vi "assignment - client.vi"() -> ()   [LabVIEW 2020]
panel:
  out "Login":bool=TRUE
  in  "Invalid":bool
  in  "stop":bool
  in  "Tab Control":T1(tab)
  in  "Enter":bool
  in  "0":bool
  in  "Reset":bool
  out "Instruction":string
  in  "9":bool
  in  "8":bool
  in  "7":bool
  in  "6":bool
  in  "5":bool
  in  "4":bool
  in  "3":bool
  in  "2":bool
  in  "1":bool
  out "PIN":string
  out "Verification":bool
  out "Time Stamp":timestamp format="%<%X\n%x>T"
  in  "Vacation mode":bool
  in  "Living Room":bool
  in  "Bedroom 1":bool
  in  "Bedroom 2":bool
  in  "Laundry 1":bool
  in  "Laundry 2":bool
  in  "Laundry 3":bool
  in  "Laundry 4":bool
  in  "Bathroom 1":bool
  in  "Bathroom 2":bool
  in  "Kitchen":bool
  in  "Dining":bool
  in  "Master":bool
  in  "Dining":dbl(knob) scale=0.0..255.0
  in  "Kitchen":dbl(knob) scale=0.0..255.0
  in  "Bathroom 2":dbl(knob) scale=0.0..255.0
  in  "Laundry 3":dbl(knob) scale=0.0..255.0
  in  "Bedroom 2":dbl(knob) scale=0.0..255.0
  in  "Bathroom 1":dbl(knob) scale=0.0..255.0
  in  "Laundry 2":dbl(knob) scale=0.0..255.0
  in  "Bedroom 1":dbl(knob) scale=0.0..255.0
  in  "Laundry 4":dbl(knob) scale=0.0..255.0
  in  "Laundry 1":dbl(knob) scale=0.0..255.0
  in  "Living Room":dbl(knob) scale=0.0..255.0
  in  "Bedroom 2":bool
  in  "Bedroom 1":bool
  in  "Master 2":bool
  in  "Automation":bool
  in  "Back":bool
  in  "Bathroom 2":bool
  in  "Laundry 4":bool
  in  "Laundry 2":bool
  in  "Laundry 1":bool
  in  "Bedroom 2":bool
  in  "Bedroom 1":bool
  in  "Front":bool
  in  "Master 3":bool
  in  "VolUp":bool
  in  "Stop":bool
  in  "Channel 2":bool
  in  "Channel 1":bool
  in  "VolDown":bool
  in  "FRwd":bool
  in  "Ffwd":bool
  in  "Pause":bool
  in  "Play":bool
  in  "Power":bool
  in  "Mute":bool
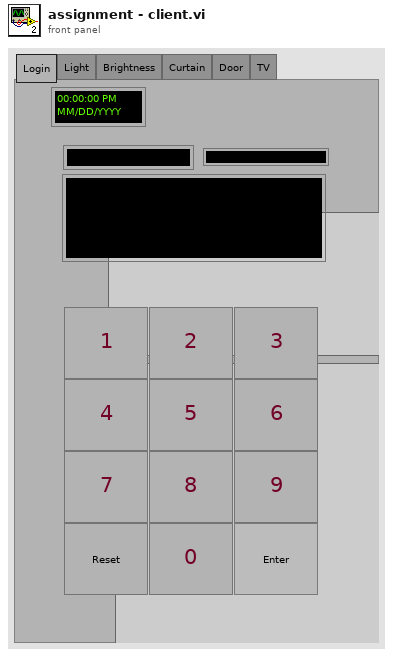
[diagram p1: front panel]
types:
  T1 = enum32{"Login", "Light", "Brightness", "Curtain", "Door", "TV"}
  T2 = enum32{"Page Enabled", "Page Disabled", "Page Disabled & Grayed"}
  T3 = enum8{"Enabled", "Disabled", "Disabled and Grayed Out"}
  T4 = enum32{"Invalid", "Standard", "Closed", "Hidden", "Minimized", "Maximized"}
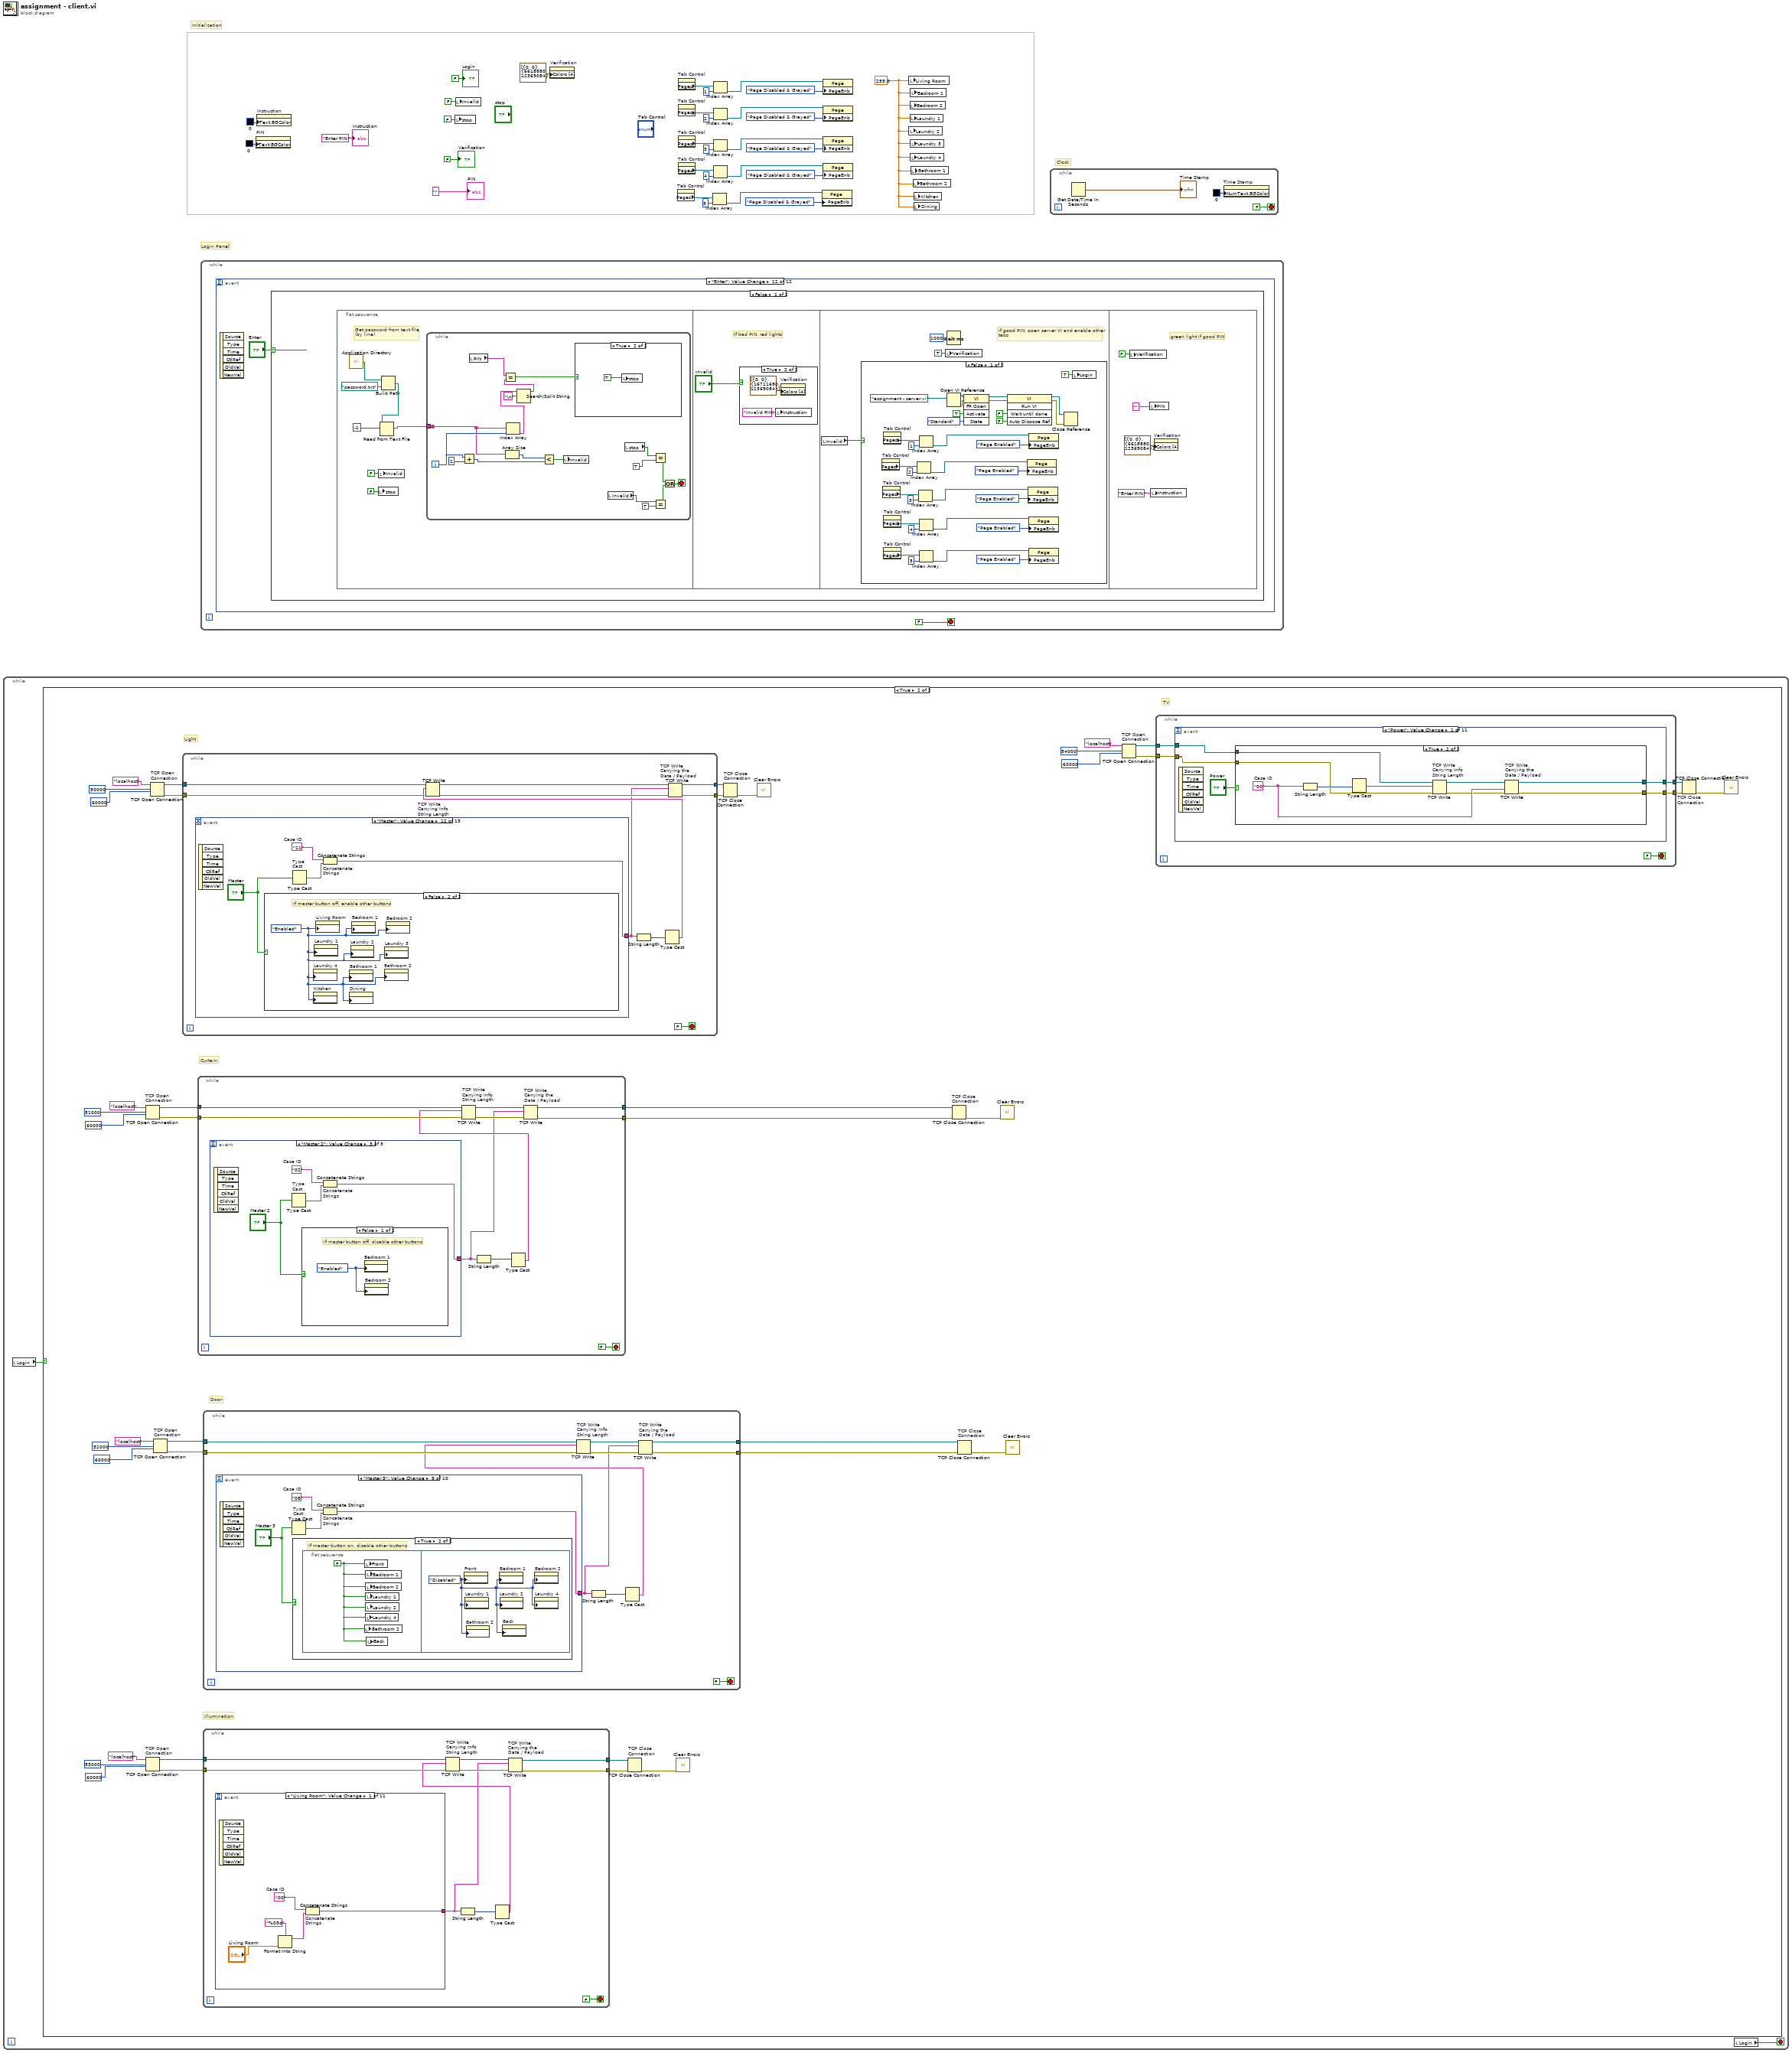
[diagram p0: block diagram]
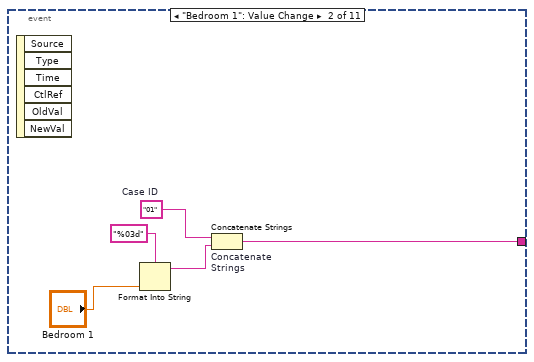
[diagram p3: hidden frame]
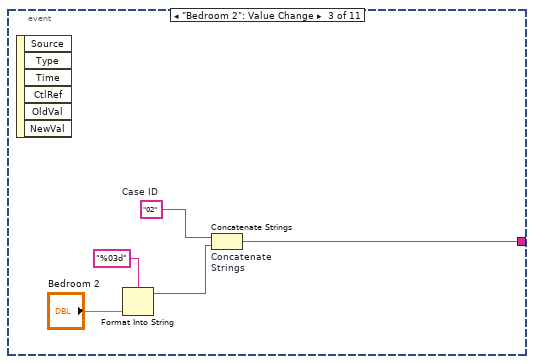
[diagram p4: hidden frame]
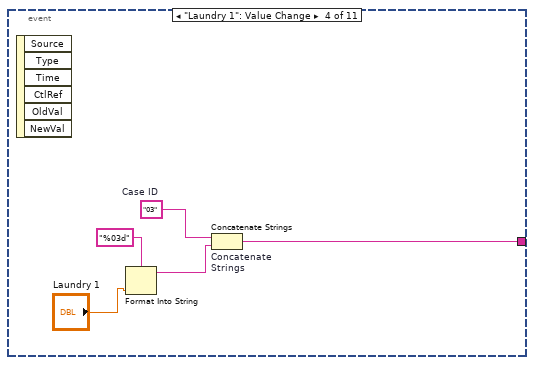
[diagram p5: hidden frame]
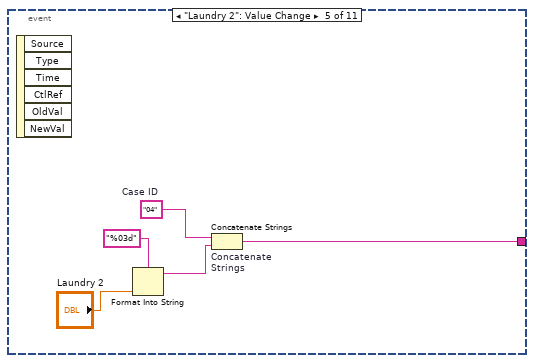
[diagram p6: hidden frame]
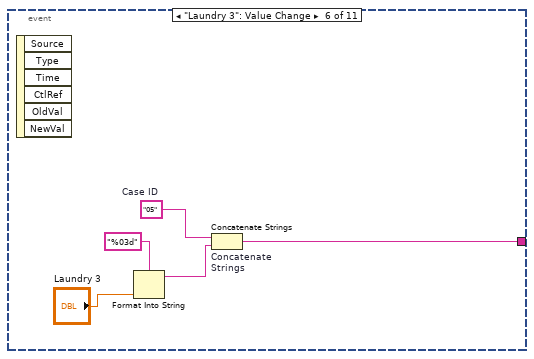
[diagram p7: hidden frame]
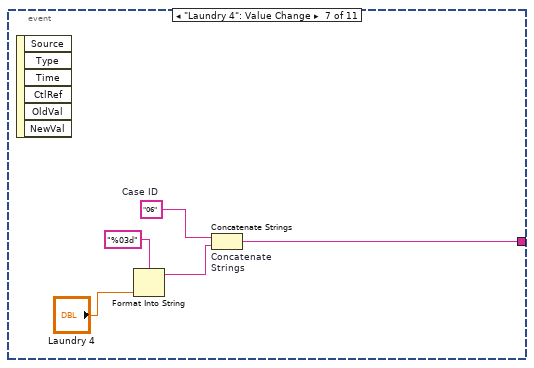
[diagram p8: hidden frame]
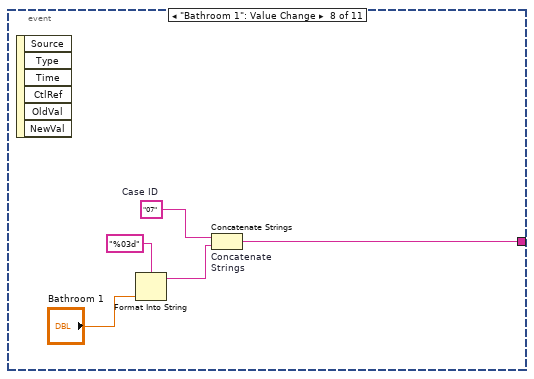
[diagram p9: hidden frame]
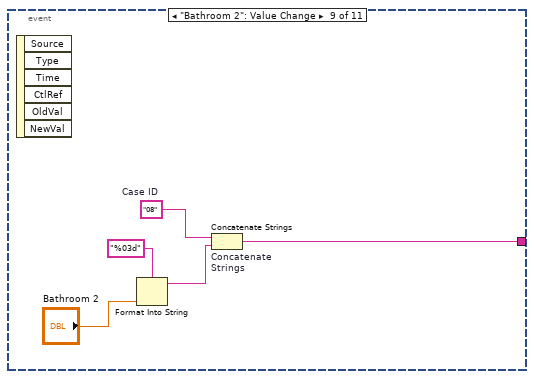
[diagram p10: hidden frame]
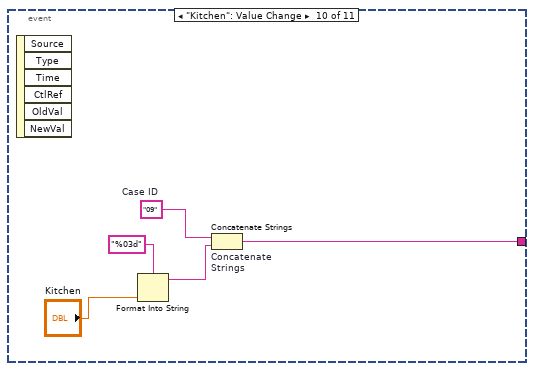
[diagram p11: hidden frame]
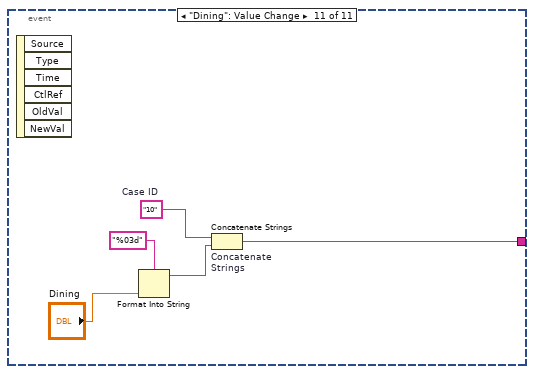
[diagram p12: hidden frame]
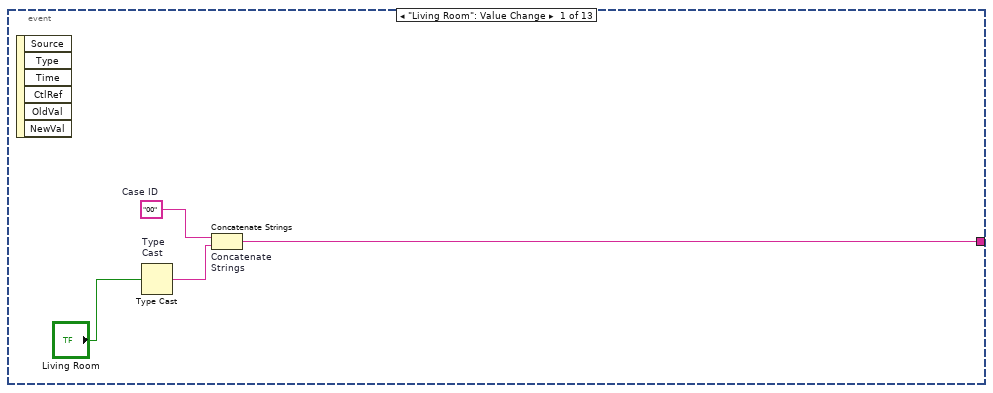
[diagram p13: hidden frame]
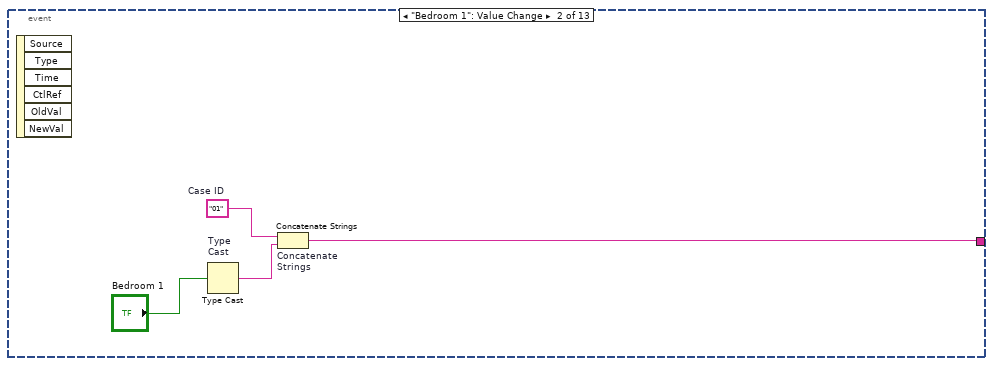
[diagram p14: hidden frame]
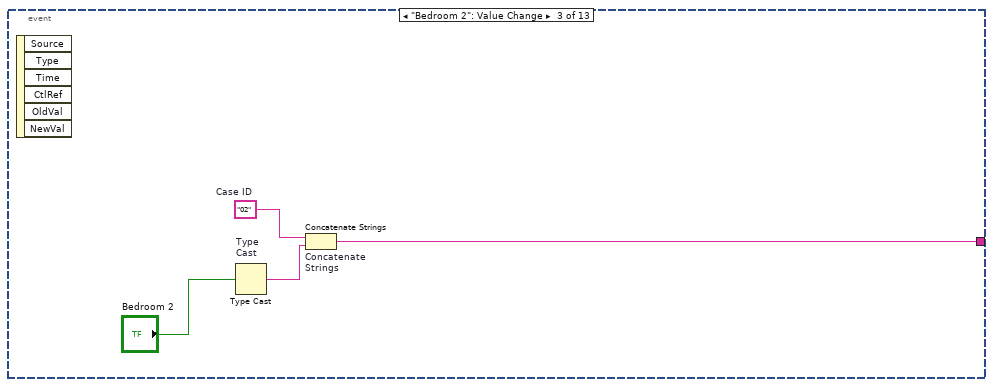
[diagram p15: hidden frame]
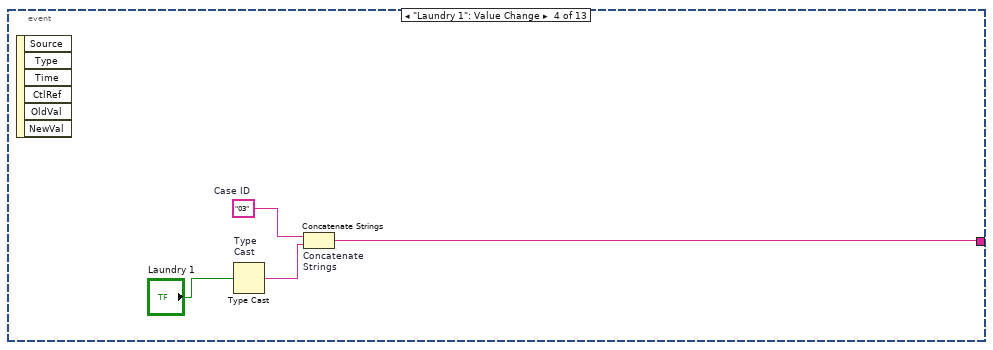
[diagram p16: hidden frame]
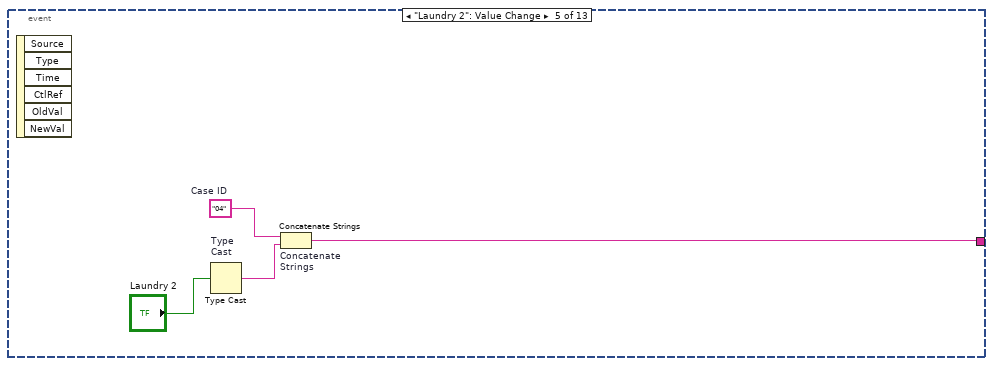
[diagram p17: hidden frame]
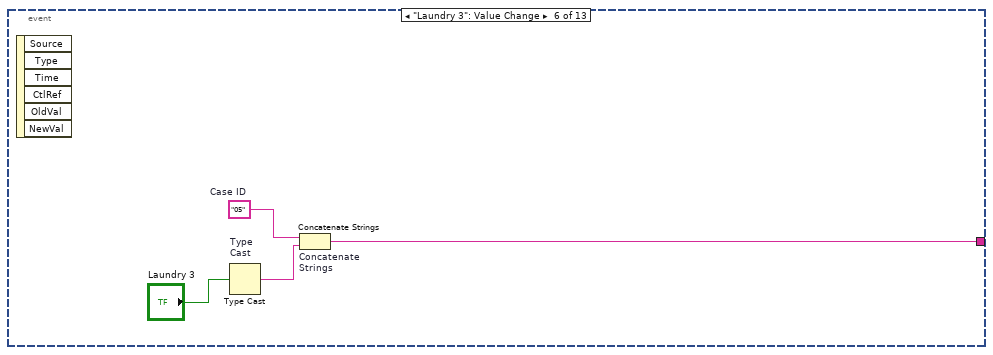
[diagram p18: hidden frame]
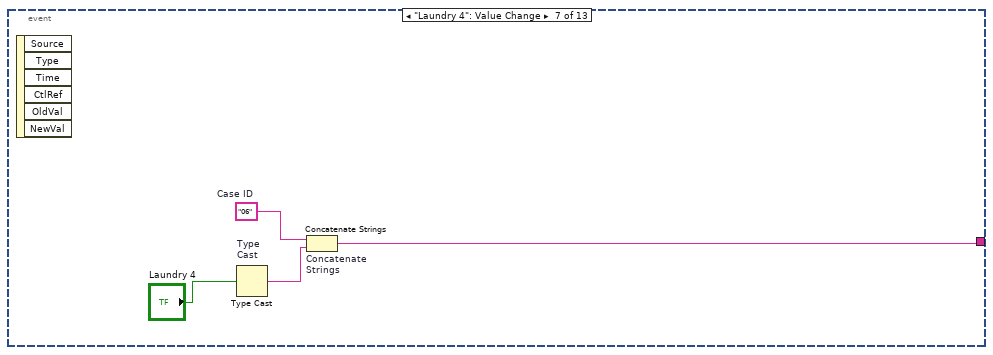
[diagram p19: hidden frame]
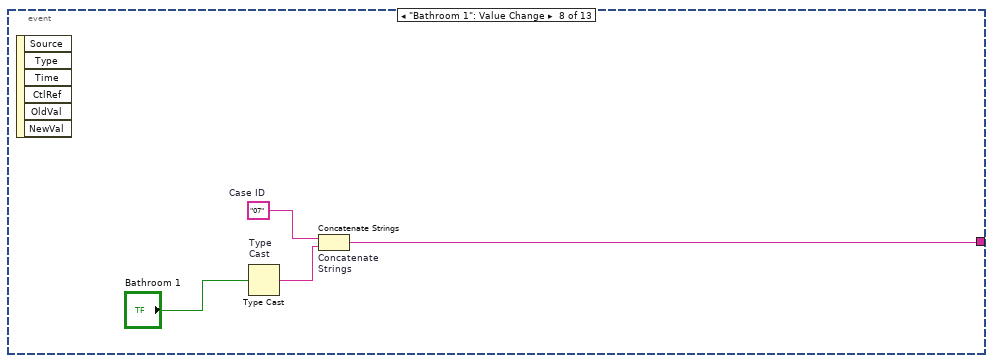
[diagram p20: hidden frame]
diagram:
  w21 = 255.0 ("Living Room")
  # "Clock"
  # "Initialization"
  # "Login Panel"
  n1 = while {
    stop <- w31 stop-if-true
    n2 = local read "Login"() -> (w32:bool)
    n3 = case shown="True" w32 {
      frame False {
      }
      frame True {
        # "TV"
        # "Illumination"
        # "Door"
        # "Curtain"
        # "Light"
        n4 = TCP Open Connection "TCP Open\nConnection"(address="localhost", remote port or service name=u16 51000, timeout ms (60000)=60000) -> (connection ID=w61:refnum<k5>, error out=w60:errorcluster)  [unwired: 2 in]
        n5 = TCP Open Connection "TCP Open\nConnection"(address="localhost", remote port or service name=u16 53000, timeout ms (60000)=60000) -> (connection ID=w33:refnum<k5>, error out=w34:errorcluster)  [unwired: 2 in]
        n6 = TCP Open Connection "TCP Open\nConnection"(address="localhost", remote port or service name=u16 50000, timeout ms (60000)=60000) -> (connection ID=w41:refnum<k5>, error out=w42:errorcluster)  [unwired: 2 in]
        n7 = TCP Open Connection "TCP Open\nConnection"(address="localhost", remote port or service name=u16 52000, timeout ms (60000)=60000) -> (connection ID=w53:refnum<k5>, error out=w52:errorcluster)  [unwired: 2 in]
        n8 = while {
          tunnel: [w141] -> w48
          tunnel: [w140] -> w47
          tunnel: w42 -> [w139]
          tunnel: w41 -> [w138]
          stop <- FALSE stop-if-true
          n9 = event shown="[11] \"Master\": Value Change" {
            selector: _ -> [_ _ _ _ _ _ _ _ _ _ _ _ _]
            dyn-events: _ -> [_ _ _ _ _ _ _ _ _ _ _ _ _]
            timeout: _ -> [_ _ _ _ _ _ _ _ _ _ _ _ _]
            tunnel: [w148 w152 w156 w161 w164 w168 w172 w176 w180 w184 w188 w193 w200] -> w142
            event "Living Room": Value Change {
              w149 = "00"  # Case ID
              n10 = event-data() -> ()  [unwired: 1 in, 6 out]
              n11 = Type Cast "Type \nCast"(x="Living Room") -> (*(type *) &x=w150:string)  [unwired: 1 in]
              n12 = Concatenate Strings "Concatenate \nStrings"(w149, w150) -> (w148:string)
            }
            event "Bedroom 1": Value Change {
              w154 = "01"  # Case ID
              n13 = event-data() -> ()  [unwired: 1 in, 6 out]
              n14 = Type Cast "Type \nCast"(x="Bedroom 1") -> (*(type *) &x=w155:string)  [unwired: 1 in]
              n15 = Concatenate Strings "Concatenate \nStrings"(w154, w155) -> (w152:string)
            }
            event "Bedroom 2": Value Change {
              w158 = "02"  # Case ID
              n16 = event-data() -> ()  [unwired: 1 in, 6 out]
              n17 = Type Cast "Type \nCast"(x="Bedroom 2") -> (*(type *) &x=w159:string)  [unwired: 1 in]
              n18 = Concatenate Strings "Concatenate \nStrings"(w158, w159) -> (w156:string)
            }
            event "Laundry 1": Value Change {
              w162 = "03"  # Case ID
              n19 = event-data() -> ()  [unwired: 1 in, 6 out]
              n20 = Type Cast "Type \nCast"(x="Laundry 1") -> (*(type *) &x=w163:string)  [unwired: 1 in]
              n21 = Concatenate Strings "Concatenate \nStrings"(w162, w163) -> (w161:string)
            }
            event "Laundry 2": Value Change {
              w166 = "04"  # Case ID
              n22 = event-data() -> ()  [unwired: 1 in, 6 out]
              n23 = Type Cast "Type \nCast"(x="Laundry 2") -> (*(type *) &x=w167:string)  [unwired: 1 in]
              n24 = Concatenate Strings "Concatenate \nStrings"(w166, w167) -> (w164:string)
            }
            event "Laundry 3": Value Change {
              w170 = "05"  # Case ID
              n25 = event-data() -> ()  [unwired: 1 in, 6 out]
              n26 = Type Cast "Type \nCast"(x="Laundry 3") -> (*(type *) &x=w171:string)  [unwired: 1 in]
              n27 = Concatenate Strings "Concatenate \nStrings"(w170, w171) -> (w168:string)
            }
            event "Laundry 4": Value Change {
              w174 = "06"  # Case ID
              n28 = event-data() -> ()  [unwired: 1 in, 6 out]
              n29 = Type Cast "Type \nCast"(x="Laundry 4") -> (*(type *) &x=w175:string)  [unwired: 1 in]
              n30 = Concatenate Strings "Concatenate \nStrings"(w174, w175) -> (w172:string)
            }
            event "Bathroom 1": Value Change {
              w178 = "07"  # Case ID
              n31 = event-data() -> ()  [unwired: 1 in, 6 out]
              n32 = Type Cast "Type \nCast"(x="Bathroom 1") -> (*(type *) &x=w179:string)  [unwired: 1 in]
              n33 = Concatenate Strings "Concatenate \nStrings"(w178, w179) -> (w176:string)
            }
            event "Bathroom 2": Value Change {
              w182 = "08"  # Case ID
              n34 = event-data() -> ()  [unwired: 1 in, 6 out]
              n35 = Type Cast "Type \nCast"(x="Bathroom 2") -> (*(type *) &x=w183:string)  [unwired: 1 in]
              n36 = Concatenate Strings "Concatenate \nStrings"(w182, w183) -> (w180:string)
            }
            event "Kitchen": Value Change {
              w186 = "09"  # Case ID
              n37 = event-data() -> ()  [unwired: 1 in, 6 out]
              n38 = Type Cast "Type \nCast"(x="Kitchen") -> (*(type *) &x=w187:string)  [unwired: 1 in]
              n39 = Concatenate Strings "Concatenate \nStrings"(w186, w187) -> (w184:string)
            }
            event "Dining": Value Change {
              w190 = "10"  # Case ID
              n40 = event-data() -> ()  [unwired: 1 in, 6 out]
              n41 = Type Cast "Type \nCast"(x="Dining") -> (*(type *) &x=w191:string)  [unwired: 1 in]
              n42 = Concatenate Strings "Concatenate \nStrings"(w190, w191) -> (w188:string)
            }
            event "Master": Value Change {
              w194 = "11"  # Case ID
              n43 = event-data() -> ()  [unwired: 1 in, 6 out]
              n44 = case shown="False" "Master" {
                frame True {
                  # "If master button ON, disable other buttons"
                  n45 = flat-sequence {
                    frame #0 {
                      w196 = FALSE ("Living Room")
                      n46 = local write "Living Room"(w196) -> ()
                      n47 = local write "Laundry 1"(w196) -> ()
                      n48 = local write "Laundry 4"(w196) -> ()
                      n49 = local write "Kitchen"(w196) -> ()
                      n50 = local write "Bedroom 1"(w196) -> ()
                      n51 = local write "Bathroom 1"(w196) -> ()
                      n52 = local write "Laundry 2"(w196) -> ()
                      n53 = local write "Dining"(w196) -> ()
                      n54 = local write "Bedroom 2"(w196) -> ()
                      n55 = local write "Laundry 3"(w196) -> ()
                      n56 = local write "Bathroom 2"(w196) -> ()
                    }
                    frame #1 {
                      w197 = T3."Disabled" ("Disabled")
                      n57 = property on="Laundry 4" class="Bool (strict)"("DisabledEnum"=w197) -> ()  [unwired: 2 in, 2 out]
                      n58 = property on="Kitchen" class="Bool (strict)"("DisabledEnum"=w197) -> ()  [unwired: 2 in, 2 out]
                      n59 = property on="Laundry 1" class="Bool (strict)"("DisabledEnum"=w197) -> ()  [unwired: 2 in, 2 out]
                      n60 = property on="Living Room" class="Bool (strict)"("DisabledEnum"=w197) -> ()  [unwired: 2 in, 2 out]
                      n61 = property on="Bathroom 1" class="Bool (strict)"("DisabledEnum"=w197) -> ()  [unwired: 2 in, 2 out]
                      n62 = property on="Dining" class="Bool (strict)"("DisabledEnum"=w197) -> ()  [unwired: 2 in, 2 out]
                      n63 = property on="Laundry 2" class="Bool (strict)"("DisabledEnum"=w197) -> ()  [unwired: 2 in, 2 out]
                      n64 = property on="Bedroom 1" class="Bool (strict)"("DisabledEnum"=w197) -> ()  [unwired: 2 in, 2 out]
                      n65 = property on="Bathroom 2" class="Bool (strict)"("DisabledEnum"=w197) -> ()  [unwired: 2 in, 2 out]
                      n66 = property on="Laundry 3" class="Bool (strict)"("DisabledEnum"=w197) -> ()  [unwired: 2 in, 2 out]
                      n67 = property on="Bedroom 2" class="Bool (strict)"("DisabledEnum"=w197) -> ()  [unwired: 2 in, 2 out]
                    }
                  }
                }
                frame False {
                  w198 = T3."Enabled" ("Disabled")
                  # "If master button off, enable other buttons"
                  n68 = property on="Laundry 4" class="Bool (strict)"("DisabledEnum"=w198) -> ()  [unwired: 2 in, 2 out]
                  n69 = property on="Kitchen" class="Bool (strict)"("DisabledEnum"=w198) -> ()  [unwired: 2 in, 2 out]
                  n70 = property on="Laundry 1" class="Bool (strict)"("DisabledEnum"=w198) -> ()  [unwired: 2 in, 2 out]
                  n71 = property on="Living Room" class="Bool (strict)"("DisabledEnum"=w198) -> ()  [unwired: 2 in, 2 out]
                  n72 = property on="Bathroom 1" class="Bool (strict)"("DisabledEnum"=w198) -> ()  [unwired: 2 in, 2 out]
                  n73 = property on="Dining" class="Bool (strict)"("DisabledEnum"=w198) -> ()  [unwired: 2 in, 2 out]
                  n74 = property on="Laundry 2" class="Bool (strict)"("DisabledEnum"=w198) -> ()  [unwired: 2 in, 2 out]
                  n75 = property on="Bedroom 1" class="Bool (strict)"("DisabledEnum"=w198) -> ()  [unwired: 2 in, 2 out]
                  n76 = property on="Bathroom 2" class="Bool (strict)"("DisabledEnum"=w198) -> ()  [unwired: 2 in, 2 out]
                  n77 = property on="Laundry 3" class="Bool (strict)"("DisabledEnum"=w198) -> ()  [unwired: 2 in, 2 out]
                  n78 = property on="Bedroom 2" class="Bool (strict)"("DisabledEnum"=w198) -> ()  [unwired: 2 in, 2 out]
                }
              }
              n79 = Type Cast "Type \nCast"(x="Master") -> (*(type *) &x=w195:string)  [unwired: 1 in]
              n80 = Concatenate Strings "Concatenate \nStrings"(w194, w195) -> (w193:string)
            }
            event "Vacation mode": Value Change {
              w201 = "12"  # Case ID
              n81 = event-data() -> ()  [unwired: 1 in, 6 out]
              n82 = Type Cast "Type \nCast"(x="Vacation mode") -> (*(type *) &x=w202:string)  [unwired: 1 in]
              n83 = Concatenate Strings "Concatenate \nStrings"(w201, w202) -> (w200:string)
            }
          }
          n84 = String Length(string=w142) -> (length=w146:i32)
          n85 = Type Cast(x=w146) -> (*(type *) &x=w145:string)  [unwired: 1 in]
          n86 = TCP Write "TCP Write\nCarrying Info\nString Length"(connection ID=w138, data in=w145, error in (no error)=w139) -> (connection ID out=w144:refnum<k5>, error out=w143:errorcluster)  [unwired: 1 in, 1 out]
          n87 = TCP Write "TCP Write\nCarrying the\nData / Payload"(connection ID=w144, data in=w142, error in (no error)=w143) -> (connection ID out=w141:refnum<k5>, error out=w140:errorcluster)  [unwired: 1 in, 1 out]
        }
        n88 = while {
          tunnel: w61 -> [w263]
          tunnel: w60 -> [w262]
          tunnel: [w257] -> w59
          tunnel: [w256] -> w58
          stop <- FALSE stop-if-true
          n89 = event shown="[2] \"Master 2\": Value Change" {
            selector: _ -> [_ _ _]
            dyn-events: _ -> [_ _ _]
            timeout: _ -> [_ _ _]
            tunnel: [w267 w271 w275] -> w258
            event "Bedroom 1": Value Change {
              w268 = "00"  # Case ID
              n90 = event-data() -> ()  [unwired: 1 in, 6 out]
              n91 = Type Cast "Type \nCast"(x="Bedroom 1") -> (*(type *) &x=w269:string)  [unwired: 1 in]
              n92 = Concatenate Strings "Concatenate \nStrings"(w268, w269) -> (w267:string)
            }
            event "Bedroom 2": Value Change {
              w272 = "01"  # Case ID
              n93 = event-data() -> ()  [unwired: 1 in, 6 out]
              n94 = Type Cast "Type \nCast"(x="Bedroom 2") -> (*(type *) &x=w273:string)  [unwired: 1 in]
              n95 = Concatenate Strings "Concatenate \nStrings"(w272, w273) -> (w271:string)
            }
            event "Master 2": Value Change {
              w276 = "02"  # Case ID
              n96 = event-data() -> ()  [unwired: 1 in, 6 out]
              n97 = Type Cast "Type \nCast"(x="Master 2") -> (*(type *) &x=w277:string)  [unwired: 1 in]
              n98 = case shown="False" "Master 2" {
                frame False {
                  w278 = T3."Enabled" ("Disabled")
                  # "If master button off, disable other buttons"
                  n99 = property on="Bedroom 1" class="Bool (strict)"("DisabledEnum"=w278) -> ()  [unwired: 2 in, 2 out]
                  n100 = property on="Bedroom 2" class="Bool (strict)"("DisabledEnum"=w278) -> ()  [unwired: 2 in, 2 out]
                }
                frame True {
                  # "If master button on, disable other buttons"
                  n101 = flat-sequence {
                    frame #0 {
                      w279 = FALSE ("Bedroom 1")
                      n102 = local write "Bedroom 1"(w279) -> ()
                      n103 = local write "Bedroom 2"(w279) -> ()
                    }
                    frame #1 {
                      w280 = T3."Disabled" ("Disabled")
                      n104 = property on="Bedroom 1" class="Bool (strict)"("DisabledEnum"=w280) -> ()  [unwired: 2 in, 2 out]
                      n105 = property on="Bedroom 2" class="Bool (strict)"("DisabledEnum"=w280) -> ()  [unwired: 2 in, 2 out]
                    }
                  }
                }
              }
              n106 = Concatenate Strings "Concatenate \nStrings"(w276, w277) -> (w275:string)
            }
          }
          n107 = String Length(string=w258) -> (length=w264:i32)
          n108 = Type Cast(x=w264) -> (*(type *) &x=w261:string)  [unwired: 1 in]
          n109 = TCP Write "TCP Write\nCarrying Info\nString Length"(connection ID=w263, data in=w261, error in (no error)=w262) -> (connection ID out=w260:refnum<k5>, error out=w259:errorcluster)  [unwired: 1 in, 1 out]
          n110 = TCP Write "TCP Write\nCarrying the\nData / Payload"(connection ID=w260, data in=w258, error in (no error)=w259) -> (connection ID out=w257:refnum<k5>, error out=w256:errorcluster)  [unwired: 1 in, 1 out]
        }
        n111 = while {
          tunnel: [w76] -> w40
          tunnel: [w75] -> w39
          tunnel: w34 -> [w74]
          tunnel: w33 -> [w73]
          stop <- FALSE stop-if-true
          n112 = event shown="[0] \"Living Room\": Value Change" {
            selector: _ -> [_ _ _ _ _ _ _ _ _ _ _]
            dyn-events: _ -> [_ _ _ _ _ _ _ _ _ _ _]
            timeout: _ -> [_ _ _ _ _ _ _ _ _ _ _]
            tunnel: [w86 w91 w96 w101 w106 w111 w116 w121 w126 w131 w136] -> w77
            event "Living Room": Value Change {
              w87 = "00"  # Case ID
              n113 = event-data() -> ()  [unwired: 1 in, 6 out]
              n114 = Format Into String "Format Into String"(format string="%03d", "Living Room") -> (resulting string=w83:string)  [unwired: 2 in, 1 out]
              n115 = Concatenate Strings "Concatenate \nStrings"(w87, w83) -> (w86:string)
            }
            event "Bedroom 1": Value Change {
              w92 = "01"  # Case ID
              n116 = event-data() -> ()  [unwired: 1 in, 6 out]
              n117 = Format Into String "Format Into String"(format string="%03d", "Bedroom 1") -> (resulting string=w88:string)  [unwired: 2 in, 1 out]
              n118 = Concatenate Strings "Concatenate \nStrings"(w92, w88) -> (w91:string)
            }
            event "Bedroom 2": Value Change {
              w97 = "02"  # Case ID
              n119 = event-data() -> ()  [unwired: 1 in, 6 out]
              n120 = Format Into String "Format Into String"(format string="%03d", "Bedroom 2") -> (resulting string=w93:string)  [unwired: 2 in, 1 out]
              n121 = Concatenate Strings "Concatenate \nStrings"(w97, w93) -> (w96:string)
            }
            event "Laundry 1": Value Change {
              w102 = "03"  # Case ID
              n122 = event-data() -> ()  [unwired: 1 in, 6 out]
              n123 = Format Into String "Format Into String"(format string="%03d", "Laundry 1") -> (resulting string=w98:string)  [unwired: 2 in, 1 out]
              n124 = Concatenate Strings "Concatenate \nStrings"(w102, w98) -> (w101:string)
            }
            event "Laundry 2": Value Change {
              w107 = "04"  # Case ID
              n125 = event-data() -> ()  [unwired: 1 in, 6 out]
              n126 = Format Into String "Format Into String"(format string="%03d", "Laundry 2") -> (resulting string=w103:string)  [unwired: 2 in, 1 out]
              n127 = Concatenate Strings "Concatenate \nStrings"(w107, w103) -> (w106:string)
            }
            event "Laundry 3": Value Change {
              w112 = "05"  # Case ID
              n128 = event-data() -> ()  [unwired: 1 in, 6 out]
              n129 = Format Into String "Format Into String"(format string="%03d", "Laundry 3") -> (resulting string=w108:string)  [unwired: 2 in, 1 out]
              n130 = Concatenate Strings "Concatenate \nStrings"(w112, w108) -> (w111:string)
            }
            event "Laundry 4": Value Change {
              w117 = "06"  # Case ID
              n131 = event-data() -> ()  [unwired: 1 in, 6 out]
              n132 = Format Into String "Format Into String"(format string="%03d", "Laundry 4") -> (resulting string=w113:string)  [unwired: 2 in, 1 out]
              n133 = Concatenate Strings "Concatenate \nStrings"(w117, w113) -> (w116:string)
            }
            event "Bathroom 1": Value Change {
              w122 = "07"  # Case ID
              n134 = event-data() -> ()  [unwired: 1 in, 6 out]
              n135 = Format Into String "Format Into String"(format string="%03d", "Bathroom 1") -> (resulting string=w118:string)  [unwired: 2 in, 1 out]
              n136 = Concatenate Strings "Concatenate \nStrings"(w122, w118) -> (w121:string)
            }
            event "Bathroom 2": Value Change {
              w127 = "08"  # Case ID
              n137 = event-data() -> ()  [unwired: 1 in, 6 out]
              n138 = Format Into String "Format Into String"(format string="%03d", "Bathroom 2") -> (resulting string=w123:string)  [unwired: 2 in, 1 out]
              n139 = Concatenate Strings "Concatenate \nStrings"(w127, w123) -> (w126:string)
            }
            event "Kitchen": Value Change {
              w132 = "09"  # Case ID
              n140 = event-data() -> ()  [unwired: 1 in, 6 out]
              n141 = Format Into String "Format Into String"(format string="%03d", "Kitchen") -> (resulting string=w128:string)  [unwired: 2 in, 1 out]
              n142 = Concatenate Strings "Concatenate \nStrings"(w132, w128) -> (w131:string)
            }
            event "Dining": Value Change {
              w137 = "10"  # Case ID
              n143 = event-data() -> ()  [unwired: 1 in, 6 out]
              n144 = Format Into String "Format Into String"(format string="%03d", "Dining") -> (resulting string=w133:string)  [unwired: 2 in, 1 out]
              n145 = Concatenate Strings "Concatenate \nStrings"(w137, w133) -> (w136:string)
            }
          }
          n146 = String Length(string=w77) -> (length=w81:i32)
          n147 = Type Cast(x=w81) -> (*(type *) &x=w80:string)  [unwired: 1 in]
          n148 = TCP Write "TCP Write\nCarrying Info\nString Length"(connection ID=w73, data in=w80, error in (no error)=w74) -> (connection ID out=w79:refnum<k5>, error out=w78:errorcluster)  [unwired: 1 in, 1 out]
          n149 = TCP Write "TCP Write\nCarrying the\nData / Payload"(connection ID=w79, data in=w77, error in (no error)=w78) -> (connection ID out=w76:refnum<k5>, error out=w75:errorcluster)  [unwired: 1 in, 1 out]
        }
        n150 = while {
          tunnel: w53 -> [w210]
          tunnel: w52 -> [w209]
          tunnel: [w204] -> w51
          tunnel: [w203] -> w50
          stop <- FALSE stop-if-true
          n151 = event shown="[8] \"Master 3\": Value Change" {
            selector: _ -> [_ _ _ _ _ _ _ _ _ _]
            dyn-events: _ -> [_ _ _ _ _ _ _ _ _ _]
            timeout: _ -> [_ _ _ _ _ _ _ _ _ _]
            tunnel: [w214 w218 w222 w226 w230 w234 w238 w242 w246 w253] -> w205
            event "Front": Value Change {
              w215 = "00"  # Case ID
              n152 = event-data() -> ()  [unwired: 1 in, 6 out]
              n153 = Type Cast "Type \nCast"(x="Front") -> (*(type *) &x=w216:string)  [unwired: 1 in]
              n154 = Concatenate Strings "Concatenate \nStrings"(w215, w216) -> (w214:string)
            }
            event "Bedroom 1": Value Change {
              w219 = "01"  # Case ID
              n155 = event-data() -> ()  [unwired: 1 in, 6 out]
              n156 = Type Cast "Type \nCast"(x="Bedroom 1") -> (*(type *) &x=w220:string)  [unwired: 1 in]
              n157 = Concatenate Strings "Concatenate \nStrings"(w219, w220) -> (w218:string)
            }
            event "Bedroom 2": Value Change {
              w223 = "02"  # Case ID
              n158 = event-data() -> ()  [unwired: 1 in, 6 out]
              n159 = Type Cast "Type \nCast"(x="Bedroom 2") -> (*(type *) &x=w224:string)  [unwired: 1 in]
              n160 = Concatenate Strings "Concatenate \nStrings"(w223, w224) -> (w222:string)
            }
            event "Laundry 1": Value Change {
              w227 = "03"  # Case ID
              n161 = event-data() -> ()  [unwired: 1 in, 6 out]
              n162 = Type Cast "Type \nCast"(x="Laundry 1") -> (*(type *) &x=w228:string)  [unwired: 1 in]
              n163 = Concatenate Strings "Concatenate \nStrings"(w227, w228) -> (w226:string)
            }
            event "Laundry 2": Value Change {
              w231 = "04"  # Case ID
              n164 = event-data() -> ()  [unwired: 1 in, 6 out]
              n165 = Type Cast "Type \nCast"(x="Laundry 2") -> (*(type *) &x=w232:string)  [unwired: 1 in]
              n166 = Concatenate Strings "Concatenate \nStrings"(w231, w232) -> (w230:string)
            }
            event "Laundry 4": Value Change {
              w235 = "05"  # Case ID
              n167 = event-data() -> ()  [unwired: 1 in, 6 out]
              n168 = Type Cast "Type \nCast"(x="Laundry 4") -> (*(type *) &x=w236:string)  [unwired: 1 in]
              n169 = Concatenate Strings "Concatenate \nStrings"(w235, w236) -> (w234:string)
            }
            event "Bathroom 2": Value Change {
              w239 = "06"  # Case ID
              n170 = event-data() -> ()  [unwired: 1 in, 6 out]
              n171 = Type Cast "Type \nCast"(x="Bathroom 2") -> (*(type *) &x=w240:string)  [unwired: 1 in]
              n172 = Concatenate Strings "Concatenate \nStrings"(w239, w240) -> (w238:string)
            }
            event "Back": Value Change {
              w243 = "07"  # Case ID
              n173 = event-data() -> ()  [unwired: 1 in, 6 out]
              n174 = Type Cast "Type \nCast"(x="Back") -> (*(type *) &x=w244:string)  [unwired: 1 in]
              n175 = Concatenate Strings "Concatenate \nStrings"(w243, w244) -> (w242:string)
            }
            event "Master 3": Value Change {
              w247 = "08"  # Case ID
              n176 = event-data() -> ()  [unwired: 1 in, 6 out]
              n177 = Type Cast "Type \nCast"(x="Master 3") -> (*(type *) &x=w248:string)  [unwired: 1 in]
              n178 = case shown="True" "Master 3" {
                frame False {
                  w249 = T3."Enabled" ("Disabled")
                  # "If master button off, disable other buttons"
                  n179 = property on="Front" class="Bool (strict)"("DisabledEnum"=w249) -> ()  [unwired: 2 in, 2 out]
                  n180 = property on="Laundry 1" class="Bool (strict)"("DisabledEnum"=w249) -> ()  [unwired: 2 in, 2 out]
                  n181 = property on="Bathroom 2" class="Bool (strict)"("DisabledEnum"=w249) -> ()  [unwired: 2 in, 2 out]
                  n182 = property on="Bedroom 1" class="Bool (strict)"("DisabledEnum"=w249) -> ()  [unwired: 2 in, 2 out]
                  n183 = property on="Laundry 2" class="Bool (strict)"("DisabledEnum"=w249) -> ()  [unwired: 2 in, 2 out]
                  n184 = property on="Back" class="Bool (strict)"("DisabledEnum"=w249) -> ()  [unwired: 2 in, 2 out]
                  n185 = property on="Bedroom 2" class="Bool (strict)"("DisabledEnum"=w249) -> ()  [unwired: 2 in, 2 out]
                  n186 = property on="Laundry 4" class="Bool (strict)"("DisabledEnum"=w249) -> ()  [unwired: 2 in, 2 out]
                }
                frame True {
                  # "If master button on, disable other buttons"
                  n187 = flat-sequence {
                    frame #0 {
                      w250 = FALSE ("Front")
                      n188 = local write "Bathroom 2"(w250) -> ()
                      n189 = local write "Front"(w250) -> ()
                      n190 = local write "Laundry 4"(w250) -> ()
                      n191 = local write "Bedroom 1"(w250) -> ()
                      n192 = local write "Bedroom 2"(w250) -> ()
                      n193 = local write "Laundry 1"(w250) -> ()
                      n194 = local write "Laundry 2"(w250) -> ()
                      n195 = local write "Back"(w250) -> ()
                    }
                    frame #1 {
                      w251 = T3."Disabled" ("Disabled")
                      n196 = property on="Front" class="Bool (strict)"("DisabledEnum"=w251) -> ()  [unwired: 2 in, 2 out]
                      n197 = property on="Laundry 1" class="Bool (strict)"("DisabledEnum"=w251) -> ()  [unwired: 2 in, 2 out]
                      n198 = property on="Bathroom 2" class="Bool (strict)"("DisabledEnum"=w251) -> ()  [unwired: 2 in, 2 out]
                      n199 = property on="Bedroom 1" class="Bool (strict)"("DisabledEnum"=w251) -> ()  [unwired: 2 in, 2 out]
                      n200 = property on="Laundry 2" class="Bool (strict)"("DisabledEnum"=w251) -> ()  [unwired: 2 in, 2 out]
                      n201 = property on="Back" class="Bool (strict)"("DisabledEnum"=w251) -> ()  [unwired: 2 in, 2 out]
                      n202 = property on="Bedroom 2" class="Bool (strict)"("DisabledEnum"=w251) -> ()  [unwired: 2 in, 2 out]
                      n203 = property on="Laundry 4" class="Bool (strict)"("DisabledEnum"=w251) -> ()  [unwired: 2 in, 2 out]
                    }
                  }
                }
              }
              n204 = Concatenate Strings "Concatenate \nStrings"(w247, w248) -> (w246:string)
            }
            event "Automation": Value Change {
              w254 = "09"  # Case ID
              n205 = event-data() -> ()  [unwired: 1 in, 6 out]
              n206 = Type Cast "Type \nCast"(x="Automation") -> (*(type *) &x=w255:string)  [unwired: 1 in]
              n207 = Concatenate Strings "Concatenate \nStrings"(w254, w255) -> (w253:string)
            }
          }
          n208 = String Length(string=w205) -> (length=w211:i32)
          n209 = Type Cast(x=w211) -> (*(type *) &x=w208:string)  [unwired: 1 in]
          n210 = TCP Write "TCP Write\nCarrying Info\nString Length"(connection ID=w210, data in=w208, error in (no error)=w209) -> (connection ID out=w207:refnum<k5>, error out=w206:errorcluster)  [unwired: 1 in, 1 out]
          n211 = TCP Write "TCP Write\nCarrying the\nData / Payload"(connection ID=w207, data in=w205, error in (no error)=w206) -> (connection ID out=w204:refnum<k5>, error out=w203:errorcluster)  [unwired: 1 in, 1 out]
        }
        n212 = TCP Close Connection "TCP Close \nConnection"(connection ID=w40, error in (no error)=w39) -> (error out=w38:errorcluster)  [unwired: 1 in, 1 out]
        n213 = call <vilib>:"Clear Errors.vi"("error in (no error)"=w38) -> ()  [unwired: 5 in, 2 out]
        n214 = TCP Close Connection "TCP Close \nConnection"(connection ID=w48, error in (no error)=w47) -> (error out=w46:errorcluster)  [unwired: 1 in, 1 out]
        n215 = call <vilib>:"Clear Errors.vi"("error in (no error)"=w46) -> ()  [unwired: 5 in, 2 out]
        n216 = TCP Close Connection "TCP Close \nConnection"(connection ID=w59, error in (no error)=w58) -> (error out=w57:errorcluster)  [unwired: 1 in, 1 out]
        n217 = TCP Close Connection "TCP Close \nConnection"(connection ID=w51, error in (no error)=w50) -> (error out=w49:errorcluster)  [unwired: 1 in, 1 out]
        n218 = call <vilib>:"Clear Errors.vi"("error in (no error)"=w57) -> ()  [unwired: 5 in, 2 out]
        n219 = call <vilib>:"Clear Errors.vi"("error in (no error)"=w49) -> ()  [unwired: 5 in, 2 out]
        n220 = TCP Open Connection "TCP Open\nConnection"(address="localhost", remote port or service name=u16 54000, timeout ms (60000)=60000) -> (connection ID=w71:refnum<k5>, error out=w72:errorcluster)  [unwired: 2 in]
        n221 = while {
          tunnel: w71 -> [w283]
          tunnel: w72 -> [w284]
          tunnel: [w282] -> w66
          tunnel: [w281] -> w65
          stop <- FALSE stop-if-true
          n222 = event shown="[0] \"Power\": Value Change" {
            selector: _ -> [_ _ _ _ _ _ _ _ _ _ _]
            dyn-events: _ -> [_ _ _ _ _ _ _ _ _ _ _]
            timeout: _ -> [_ _ _ _ _ _ _ _ _ _ _]
            tunnel: w284 -> [w289 w306 w322 w338 w354 w370 w386 w402 w418 w434 w450]
            tunnel: w283 -> [w288 w305 w321 w337 w353 w369 w385 w401 w417 w433 w449]
            tunnel: [w287 w302 w318 w334 w350 w366 w382 w398 w414 w430 w446] -> w282
            tunnel: [w286 w303 w319 w335 w351 w367 w383 w399 w415 w431 w447] -> w281
            event "Power": Value Change {
              n223 = event-data() -> ()  [unwired: 1 in, 6 out]
              n224 = case shown="True" "Power" {
                tunnel: w289 -> [w291 w300]
                tunnel: w288 -> [w292 w299]
                tunnel: [w291 w294] -> w287
                tunnel: [w292 w293] -> w286
                frame False {
                }
                frame True {
                  w296 = "00"  # Case ID
                  n225 = String Length(string=w296) -> (length=w301:i32)
                  n226 = Type Cast(x=w301) -> (*(type *) &x=w298:string)  [unwired: 1 in]
                  n227 = TCP Write "TCP Write\nCarrying Info\nString Length"(connection ID=w299, data in=w298, error in (no error)=w300) -> (connection ID out=w297:refnum<k5>, error out=w295:errorcluster)  [unwired: 1 in, 1 out]
                  n228 = TCP Write "TCP Write\nCarrying the\nData / Payload"(connection ID=w297, data in=w296, error in (no error)=w295) -> (connection ID out=w293:refnum<k5>, error out=w294:errorcluster)  [unwired: 1 in, 1 out]
                }
              }
            }
            event "Channel 1": Value Change {
              n229 = event-data() -> ()  [unwired: 1 in, 6 out]
              n230 = case shown="True" "Channel 1" {
                tunnel: w306 -> [w307 w316]
                tunnel: w305 -> [w308 w315]
                tunnel: [w308 w310] -> w303
                tunnel: [w307 w309] -> w302
                frame False {
                }
                frame True {
                  w312 = "01"  # Case ID
                  n231 = String Length(string=w312) -> (length=w317:i32)
                  n232 = Type Cast(x=w317) -> (*(type *) &x=w314:string)  [unwired: 1 in]
                  n233 = TCP Write "TCP Write\nCarrying Info\nString Length"(connection ID=w315, data in=w314, error in (no error)=w316) -> (connection ID out=w313:refnum<k5>, error out=w311:errorcluster)  [unwired: 1 in, 1 out]
                  n234 = TCP Write "TCP Write\nCarrying the\nData / Payload"(connection ID=w313, data in=w312, error in (no error)=w311) -> (connection ID out=w310:refnum<k5>, error out=w309:errorcluster)  [unwired: 1 in, 1 out]
                }
              }
            }
            event "Channel 2": Value Change {
              n235 = event-data() -> ()  [unwired: 1 in, 6 out]
              n236 = case shown="False" "Channel 2" {
                tunnel: w322 -> [w323 w332]
                tunnel: w321 -> [w324 w331]
                tunnel: [w324 w326] -> w319
                tunnel: [w323 w325] -> w318
                frame False {
                }
                frame True {
                  w328 = "02"  # Case ID
                  n237 = String Length(string=w328) -> (length=w333:i32)
                  n238 = Type Cast(x=w333) -> (*(type *) &x=w330:string)  [unwired: 1 in]
                  n239 = TCP Write "TCP Write\nCarrying Info\nString Length"(connection ID=w331, data in=w330, error in (no error)=w332) -> (connection ID out=w329:refnum<k5>, error out=w327:errorcluster)  [unwired: 1 in, 1 out]
                  n240 = TCP Write "TCP Write\nCarrying the\nData / Payload"(connection ID=w329, data in=w328, error in (no error)=w327) -> (connection ID out=w326:refnum<k5>, error out=w325:errorcluster)  [unwired: 1 in, 1 out]
                }
              }
            }
            event "Play": Value Change {
              n241 = event-data() -> ()  [unwired: 1 in, 6 out]
              n242 = case shown="False" "Play" {
                tunnel: w338 -> [w339 w348]
                tunnel: w337 -> [w340 w347]
                tunnel: [w340 w342] -> w335
                tunnel: [w339 w341] -> w334
                frame False {
                }
                frame True {
                  w344 = "03"  # Case ID
                  n243 = String Length(string=w344) -> (length=w349:i32)
                  n244 = Type Cast(x=w349) -> (*(type *) &x=w346:string)  [unwired: 1 in]
                  n245 = TCP Write "TCP Write\nCarrying Info\nString Length"(connection ID=w347, data in=w346, error in (no error)=w348) -> (connection ID out=w345:refnum<k5>, error out=w343:errorcluster)  [unwired: 1 in, 1 out]
                  n246 = TCP Write "TCP Write\nCarrying the\nData / Payload"(connection ID=w345, data in=w344, error in (no error)=w343) -> (connection ID out=w342:refnum<k5>, error out=w341:errorcluster)  [unwired: 1 in, 1 out]
                }
              }
            }
            event "Pause": Value Change {
              n247 = event-data() -> ()  [unwired: 1 in, 6 out]
              n248 = case shown="False" "Pause" {
                tunnel: w354 -> [w355 w364]
                tunnel: w353 -> [w356 w363]
                tunnel: [w356 w358] -> w351
                tunnel: [w355 w357] -> w350
                frame False {
                }
                frame True {
                  w360 = "04"  # Case ID
                  n249 = String Length(string=w360) -> (length=w365:i32)
                  n250 = Type Cast(x=w365) -> (*(type *) &x=w362:string)  [unwired: 1 in]
                  n251 = TCP Write "TCP Write\nCarrying Info\nString Length"(connection ID=w363, data in=w362, error in (no error)=w364) -> (connection ID out=w361:refnum<k5>, error out=w359:errorcluster)  [unwired: 1 in, 1 out]
                  n252 = TCP Write "TCP Write\nCarrying the\nData / Payload"(connection ID=w361, data in=w360, error in (no error)=w359) -> (connection ID out=w358:refnum<k5>, error out=w357:errorcluster)  [unwired: 1 in, 1 out]
                }
              }
            }
            event "Stop": Value Change {
              n253 = event-data() -> ()  [unwired: 1 in, 6 out]
              n254 = case shown="False" "Stop" {
                tunnel: w370 -> [w371 w380]
                tunnel: w369 -> [w372 w379]
                tunnel: [w372 w374] -> w367
                tunnel: [w371 w373] -> w366
                frame False {
                }
                frame True {
                  w376 = "05"  # Case ID
                  n255 = String Length(string=w376) -> (length=w381:i32)
                  n256 = Type Cast(x=w381) -> (*(type *) &x=w378:string)  [unwired: 1 in]
                  n257 = TCP Write "TCP Write\nCarrying Info\nString Length"(connection ID=w379, data in=w378, error in (no error)=w380) -> (connection ID out=w377:refnum<k5>, error out=w375:errorcluster)  [unwired: 1 in, 1 out]
                  n258 = TCP Write "TCP Write\nCarrying the\nData / Payload"(connection ID=w377, data in=w376, error in (no error)=w375) -> (connection ID out=w374:refnum<k5>, error out=w373:errorcluster)  [unwired: 1 in, 1 out]
                }
              }
            }
            event "FRwd": Value Change {
              n259 = event-data() -> ()  [unwired: 1 in, 6 out]
              n260 = case shown="True" "FRwd" {
                tunnel: w386 -> [w387 w396]
                tunnel: w385 -> [w388 w395]
                tunnel: [w388 w390] -> w383
                tunnel: [w387 w389] -> w382
                frame False {
                }
                frame True {
                  w392 = "06"  # Case ID
                  n261 = String Length(string=w392) -> (length=w397:i32)
                  n262 = Type Cast(x=w397) -> (*(type *) &x=w394:string)  [unwired: 1 in]
                  n263 = TCP Write "TCP Write\nCarrying Info\nString Length"(connection ID=w395, data in=w394, error in (no error)=w396) -> (connection ID out=w393:refnum<k5>, error out=w391:errorcluster)  [unwired: 1 in, 1 out]
                  n264 = TCP Write "TCP Write\nCarrying the\nData / Payload"(connection ID=w393, data in=w392, error in (no error)=w391) -> (connection ID out=w390:refnum<k5>, error out=w389:errorcluster)  [unwired: 1 in, 1 out]
                }
              }
            }
            event "Ffwd": Value Change {
              n265 = event-data() -> ()  [unwired: 1 in, 6 out]
              n266 = case shown="True" "Ffwd" {
                tunnel: w402 -> [w403 w412]
                tunnel: w401 -> [w404 w411]
                tunnel: [w404 w406] -> w399
                tunnel: [w403 w405] -> w398
                frame False {
                }
                frame True {
                  w408 = "07"  # Case ID
                  n267 = String Length(string=w408) -> (length=w413:i32)
                  n268 = Type Cast(x=w413) -> (*(type *) &x=w410:string)  [unwired: 1 in]
                  n269 = TCP Write "TCP Write\nCarrying Info\nString Length"(connection ID=w411, data in=w410, error in (no error)=w412) -> (connection ID out=w409:refnum<k5>, error out=w407:errorcluster)  [unwired: 1 in, 1 out]
                  n270 = TCP Write "TCP Write\nCarrying the\nData / Payload"(connection ID=w409, data in=w408, error in (no error)=w407) -> (connection ID out=w406:refnum<k5>, error out=w405:errorcluster)  [unwired: 1 in, 1 out]
                }
              }
            }
            event "VolDown": Value Change {
              n271 = event-data() -> ()  [unwired: 1 in, 6 out]
              n272 = case shown="True" "VolDown" {
                tunnel: w418 -> [w419 w428]
                tunnel: w417 -> [w420 w427]
                tunnel: [w420 w422] -> w415
                tunnel: [w419 w421] -> w414
                frame False {
                }
                frame True {
                  w424 = "10"  # Case ID
                  n273 = String Length(string=w424) -> (length=w429:i32)
                  n274 = Type Cast(x=w429) -> (*(type *) &x=w426:string)  [unwired: 1 in]
                  n275 = TCP Write "TCP Write\nCarrying Info\nString Length"(connection ID=w427, data in=w426, error in (no error)=w428) -> (connection ID out=w425:refnum<k5>, error out=w423:errorcluster)  [unwired: 1 in, 1 out]
                  n276 = TCP Write "TCP Write\nCarrying the\nData / Payload"(connection ID=w425, data in=w424, error in (no error)=w423) -> (connection ID out=w422:refnum<k5>, error out=w421:errorcluster)  [unwired: 1 in, 1 out]
                }
              }
            }
            event "VolUp": Value Change {
              n277 = event-data() -> ()  [unwired: 1 in, 6 out]
              n278 = case shown="True" "VolUp" {
                tunnel: w434 -> [w435 w444]
                tunnel: w433 -> [w436 w443]
                tunnel: [w436 w438] -> w431
                tunnel: [w435 w437] -> w430
                frame False {
                }
                frame True {
                  w440 = "11"  # Case ID
                  n279 = String Length(string=w440) -> (length=w445:i32)
                  n280 = Type Cast(x=w445) -> (*(type *) &x=w442:string)  [unwired: 1 in]
                  n281 = TCP Write "TCP Write\nCarrying Info\nString Length"(connection ID=w443, data in=w442, error in (no error)=w444) -> (connection ID out=w441:refnum<k5>, error out=w439:errorcluster)  [unwired: 1 in, 1 out]
                  n282 = TCP Write "TCP Write\nCarrying the\nData / Payload"(connection ID=w441, data in=w440, error in (no error)=w439) -> (connection ID out=w438:refnum<k5>, error out=w437:errorcluster)  [unwired: 1 in, 1 out]
                }
              }
            }
            event "Mute": Value Change {
              n283 = event-data() -> ()  [unwired: 1 in, 6 out]
              n284 = case shown="False" "Mute" {
                tunnel: w450 -> [w451 w460]
                tunnel: w449 -> [w452 w459]
                tunnel: [w452 w454] -> w447
                tunnel: [w451 w453] -> w446
                frame False {
                }
                frame True {
                  w456 = "12"  # Case ID
                  n285 = String Length(string=w456) -> (length=w461:i32)
                  n286 = Type Cast(x=w461) -> (*(type *) &x=w458:string)  [unwired: 1 in]
                  n287 = TCP Write "TCP Write\nCarrying Info\nString Length"(connection ID=w459, data in=w458, error in (no error)=w460) -> (connection ID out=w457:refnum<k5>, error out=w455:errorcluster)  [unwired: 1 in, 1 out]
                  n288 = TCP Write "TCP Write\nCarrying the\nData / Payload"(connection ID=w457, data in=w456, error in (no error)=w455) -> (connection ID out=w454:refnum<k5>, error out=w453:errorcluster)  [unwired: 1 in, 1 out]
                }
              }
            }
          }
        }
        n289 = TCP Close Connection "TCP Close \nConnection"(connection ID=w65, error in (no error)=w66) -> (error out=w67:errorcluster)  [unwired: 1 in, 1 out]
        n290 = call <vilib>:"Clear Errors.vi"("error in (no error)"=w67) -> ()  [unwired: 5 in, 2 out]
      }
    }
    n291 = local read "Login"() -> (w31:bool)
  }
  n292 = while {
    stop <- FALSE stop-if-true
    n293 = event shown="[11] \"Enter\": Value Change" {
      selector: _ -> [_ _ _ _ _ _ _ _ _ _ _ _]
      dyn-events: _ -> [_ _ _ _ _ _ _ _ _ _ _ _]
      timeout: _ -> [_ _ _ _ _ _ _ _ _ _ _ _]
      event "1": Value Change {
        n294 = event-data() -> ()  [unwired: 1 in, 6 out]
        n295 = case shown="True" "1" {
          frame False {
            n296 = local read "PIN"() -> (w467:string)
            n297 = String Length(string=w467) -> (length=w466:i32)
            n298 = Less?(x=w466, y=4) -> (x < y?=w464:bool)
            n299 = case shown="True" w464 {
              frame False {
              }
              frame True {
                n300 = local read "PIN"() -> (w470:string)
                n301 = Concatenate Strings(w470, "1" ("string")) -> (w468:string)
                n302 = local write "PIN"(w468) -> ()
              }
            }
          }
          frame True {
          }
        }
      }
      event "2": Value Change {
        n303 = event-data() -> ()  [unwired: 1 in, 6 out]
        n304 = case shown="False" "2" {
          frame False {
            n305 = local read "PIN"() -> (w475:string)
            n306 = String Length(string=w475) -> (length=w474:i32)
            n307 = Less?(x=w474, y=4) -> (x < y?=w472:bool)
            n308 = case shown="True" w472 {
              frame False {
              }
              frame True {
                n309 = local read "PIN"() -> (w478:string)
                n310 = Concatenate Strings "Concatenate Strings"(w478, "2" ("string")) -> (w476:string)
                n311 = local write "PIN"(w476) -> ()
              }
            }
          }
          frame True {
          }
        }
      }
      event "3": Value Change {
        n312 = event-data() -> ()  [unwired: 1 in, 6 out]
        n313 = case shown="True" "3" {
          frame False {
          }
          frame True {
            n314 = local read "PIN"() -> (w483:string)
            n315 = String Length(string=w483) -> (length=w482:i32)
            n316 = Less?(x=w482, y=4) -> (x < y?=w480:bool)
            n317 = case shown="True" w480 {
              frame False {
              }
              frame True {
                n318 = local read "PIN"() -> (w486:string)
                n319 = Concatenate Strings "Concatenate Strings"(w486, "3" ("string")) -> (w484:string)
                n320 = local write "PIN"(w484) -> ()
              }
            }
          }
        }
      }
      event "4": Value Change {
        n321 = event-data() -> ()  [unwired: 1 in, 6 out]
        n322 = case shown="False" "4" {
          frame False {
            n323 = local read "PIN"() -> (w491:string)
            n324 = String Length(string=w491) -> (length=w490:i32)
            n325 = Less?(x=w490, y=4) -> (x < y?=w488:bool)
            n326 = case shown="True" w488 {
              frame False {
              }
              frame True {
                n327 = local read "PIN"() -> (w494:string)
                n328 = Concatenate Strings "Concatenate Strings"(w494, "4" ("string")) -> (w492:string)
                n329 = local write "PIN"(w492) -> ()
              }
            }
          }
          frame True {
          }
        }
      }
      event "5": Value Change {
        n330 = event-data() -> ()  [unwired: 1 in, 6 out]
        n331 = case shown="False" "5" {
          frame False {
            n332 = local read "PIN"() -> (w499:string)
            n333 = String Length(string=w499) -> (length=w498:i32)
            n334 = Less?(x=w498, y=4) -> (x < y?=w496:bool)
            n335 = case shown="True" w496 {
              frame False {
              }
              frame True {
                n336 = local read "PIN"() -> (w502:string)
                n337 = Concatenate Strings "Concatenate Strings"(w502, "5" ("string")) -> (w500:string)
                n338 = local write "PIN"(w500) -> ()
              }
            }
          }
          frame True {
          }
        }
      }
      event "6": Value Change {
        n339 = event-data() -> ()  [unwired: 1 in, 6 out]
        n340 = case shown="False" "6" {
          frame False {
            n341 = local read "PIN"() -> (w507:string)
            n342 = String Length(string=w507) -> (length=w506:i32)
            n343 = Less?(x=w506, y=4) -> (x < y?=w504:bool)
            n344 = case shown="True" w504 {
              frame False {
              }
              frame True {
                n345 = local read "PIN"() -> (w510:string)
                n346 = Concatenate Strings "Concatenate Strings"(w510, "6" ("string")) -> (w508:string)
                n347 = local write "PIN"(w508) -> ()
              }
            }
          }
          frame True {
          }
        }
      }
      event "7": Value Change {
        n348 = event-data() -> ()  [unwired: 1 in, 6 out]
        n349 = case shown="False" "7" {
          frame False {
            n350 = local read "PIN"() -> (w515:string)
            n351 = String Length(string=w515) -> (length=w514:i32)
            n352 = Less?(x=w514, y=4) -> (x < y?=w512:bool)
            n353 = case shown="True" w512 {
              frame False {
              }
              frame True {
                n354 = local read "PIN"() -> (w518:string)
                n355 = Concatenate Strings "Concatenate Strings"(w518, "7" ("string")) -> (w516:string)
                n356 = local write "PIN"(w516) -> ()
              }
            }
          }
          frame True {
          }
        }
      }
      event "8": Value Change {
        n357 = event-data() -> ()  [unwired: 1 in, 6 out]
        n358 = case shown="False" "8" {
          frame False {
            n359 = local read "PIN"() -> (w523:string)
            n360 = String Length(string=w523) -> (length=w522:i32)
            n361 = Less?(x=w522, y=4) -> (x < y?=w520:bool)
            n362 = case shown="True" w520 {
              frame False {
              }
              frame True {
                n363 = local read "PIN"() -> (w526:string)
                n364 = Concatenate Strings "Concatenate Strings"(w526, "8" ("string")) -> (w524:string)
                n365 = local write "PIN"(w524) -> ()
              }
            }
          }
          frame True {
          }
        }
      }
      event "9": Value Change {
        n366 = event-data() -> ()  [unwired: 1 in, 6 out]
        n367 = case shown="False" "9" {
          frame False {
            n368 = local read "PIN"() -> (w531:string)
            n369 = String Length(string=w531) -> (length=w530:i32)
            n370 = Less?(x=w530, y=4) -> (x < y?=w528:bool)
            n371 = case shown="True" w528 {
              frame False {
              }
              frame True {
                n372 = local read "PIN"() -> (w534:string)
                n373 = Concatenate Strings "Concatenate Strings"(w534, "9" ("string")) -> (w532:string)
                n374 = local write "PIN"(w532) -> ()
              }
            }
          }
          frame True {
          }
        }
      }
      event "0": Value Change {
        n375 = event-data() -> ()  [unwired: 1 in, 6 out]
        n376 = case shown="False" "0" {
          frame False {
            n377 = local read "PIN"() -> (w539:string)
            n378 = String Length(string=w539) -> (length=w538:i32)
            n379 = Less?(x=w538, y=4) -> (x < y?=w536:bool)
            n380 = case shown="True" w536 {
              frame False {
              }
              frame True {
                n381 = local read "PIN"() -> (w542:string)
                n382 = Concatenate Strings "Concatenate Strings"(w542, "0" ("string")) -> (w540:string)
                n383 = local write "PIN"(w540) -> ()
              }
            }
          }
          frame True {
          }
        }
      }
      event "Reset": Value Change {
        n384 = event-data() -> ()  [unwired: 1 in, 6 out]
        n385 = case shown="False" "Reset" {
          frame False {
            n386 = local write "PIN"("" ("PIN")) -> ()
          }
          frame True {
          }
        }
      }
      event "Enter": Value Change {
        n387 = event-data() -> ()  [unwired: 1 in, 6 out]
        n388 = case shown="False" "Enter" {
          frame False {
            n389 = flat-sequence {
              frame #0 {
                # "Get password from text file\n(by line)"
                n390 = call <vilib>:"Application Directory.vi"() -> ("Application Directory"=w546:path)
                n391 = local write "stop"(FALSE ("stop")) -> ()
                n392 = local write "Invalid"(FALSE ("Invalid")) -> ()
                n393 = Build Path(base path=w546, name or relative path=path "password.txt") -> (appended path=w547:path)
                n394 = Read from Text File(file (use dialog)=w547, count=-1) -> (text=w551:string[])  [unwired: 2 in, 3 out]
                n395 = while {
                  tunnel: [w558] -> _
                  tunnel: w551 -> [w558]
                  i -> [w567]
                  stop <- w553 stop-if-true
                  n396 = Add(x=w567, y=1) -> (x+y=w564:i32)
                  n397 = local read "PIN"() -> (w570:string)
                  n398 = Array Size(array=w558) -> (size(s)=w565:i32)
                  n399 = Index Array "Index Array"(array=w558, index=w567) -> (element=w562:string)
                  n400 = Search/Split String(string=w562, search string/char (-)="\n") -> (substring before match=w560:string)  [unwired: 1 in, 2 out]
                  n401 = Equal?(x=w570, y=w560) -> (x = y?=w569:bool)
                  n402 = Less?(x=w565, y=w564) -> (x < y?=w563:bool)
                  n403 = local write "Invalid"(w563) -> ()
                  n404 = case shown="True" w569 {
                    frame False {
                    }
                    frame True {
                      n405 = local write "stop"(TRUE ("Verification")) -> ()
                    }
                  }
                  n406 = local read "Invalid"() -> (w555:bool)
                  n407 = local read "stop"() -> (w559:bool)
                  n408 = Equal?(x=w559, y=TRUE) -> (x = y?=w557:bool)
                  n409 = Equal?(x=w555, y=TRUE) -> (x = y?=w556:bool)
                  n410 = Or(x=w557, y=w556) -> (x .or. y?=w553:bool)
                }
              }
              frame #1 {
                # "If bad PIN, red lights"
                n411 = case shown="True" "Invalid" {
                  frame False {
                  }
                  frame True {
                    n412 = local write "Instruction"("Invalid PIN" ("Instruction")) -> ()
                    n413 = property on="Verification" class="Bool (strict)"("Colors [4]"=cluster{u32, u32}[] [{0, 0}, {16711680, 12369084}]) -> ()  [unwired: 2 in, 2 out]
                  }
                }
              }
              frame #2 {
                # "If good PIN, open server VI and enable other\ntabs"
                n414 = local read "Invalid"() -> (w575:bool)
                n415 = case shown="False" w575 {
                  frame False {
                    n416 = property on="Tab Control" class="TabCtl (strict)"() -> ("Pages"=w590:refnum<vi>[])  [unwired: 2 in, 2 out]
                    n417 = property on="Tab Control" class="TabCtl (strict)"() -> ("Pages"=w589:refnum<vi>[])  [unwired: 2 in, 2 out]
                    n418 = property on="Tab Control" class="TabCtl (strict)"() -> ("Pages"=w597:refnum<vi>[])  [unwired: 2 in, 2 out]
                    n419 = property on="Tab Control" class="TabCtl (strict)"() -> ("Pages"=w582:refnum<vi>[])  [unwired: 2 in, 2 out]
                    n420 = property on="Tab Control" class="TabCtl (strict)"() -> ("Pages"=w581:refnum<vi>[])  [unwired: 2 in, 2 out]
                    n421 = Index Array(array=w590, index=2) -> (element=w591:refnum<vi>)
                    n422 = Index Array(array=w589, index=3) -> (element=w588:refnum<vi>)
                    n423 = Index Array(array=w597, index=1) -> (element=w596:refnum<vi>)
                    n424 = Index Array(array=w582, index=4) -> (element=w583:refnum<vi>)
                    n425 = Index Array(array=w581, index=5) -> (element=w580:refnum<vi>)
                    n426 = Open VI Reference(vi path=path "assignment - server.vi") -> (vi reference=w608:refnum<vi>, error out=w607:errorcluster)  [unwired: 5 in]
                    n427 = invoke class="VI" method="FP.Open"(reference=w608, error in=w607, "Activate"=TRUE ("Activate?"), "State"=T4."Standard") -> (reference out=w606:refnum<vi>, error out=w605:errorcluster)  [unwired: 1 in, 3 out]
                    n428 = invoke class="VI" method="Run VI"(reference=w606, error in=w605, "Wait until done"=FALSE ("Wait Until Done"), "Auto Dispose Ref"=FALSE ("Auto Dispose Reference")) -> (reference out=w600:refnum<vi>, error out=w599:errorcluster)  [unwired: 1 in, 3 out]
                    n429 = property class="Page"(reference=w591, "PageEnb"=T2."Page Enabled" ("Page Enabled State")) -> ()  [unwired: 1 in, 2 out]
                    n430 = property class="Page"(reference=w588, "PageEnb"=T2."Page Enabled" ("Page Enabled State")) -> ()  [unwired: 1 in, 2 out]
                    n431 = property class="Page"(reference=w596, "PageEnb"=T2."Page Enabled" ("Page Enabled State")) -> ()  [unwired: 1 in, 2 out]
                    n432 = property class="Page"(reference=w583, "PageEnb"=T2."Page Enabled" ("Page Enabled State")) -> ()  [unwired: 1 in, 2 out]
                    n433 = property class="Page"(reference=w580, "PageEnb"=T2."Page Enabled" ("Page Enabled State")) -> ()  [unwired: 1 in, 2 out]
                    n434 = Close Reference(reference=w600, error in (no error)=w599) -> ()  [unwired: 1 out]
                    n435 = local write "Login"(TRUE ("Login")) -> ()
                  }
                  frame True {
                  }
                }
                n436 = local write "Verification"(TRUE ("Verification")) -> ()
                n437 = Wait (ms)(milliseconds to wait=u32 1000) -> ()  [unwired: 1 out]
              }
              frame #3 {
                # "green light if good PIN"
                n438 = local write "Verification"(FALSE ("Verification")) -> ()
                n439 = local write "PIN"("" ("PIN")) -> ()
                n440 = local write "Instruction"("Enter PIN:" ("Instruction")) -> ()
                n441 = property on="Verification" class="Bool (strict)"("Colors [4]"=cluster{u32, u32}[] [{0, 0}, {6618880, 12369084}]) -> ()  [unwired: 2 in, 2 out]
              }
            }
          }
          frame True {
          }
        }
      }
    }
  }
  n442 = property on="PIN" class="Str"("Text.BGColor"=u32 0 ("Text.Text Colors:BG Color")) -> ()  [unwired: 2 in, 2 out]
  n443 = property on="Instruction" class="Str"("Text.BGColor"=u32 0 ("Text.Text Colors:BG Color")) -> ()  [unwired: 2 in, 2 out]
  n444 = local write "stop"(FALSE ("stop")) -> ()
  n445 = local write "Invalid"(FALSE ("Invalid")) -> ()
  n446 = property on="Verification" class="Bool (strict)"("Colors [4]"=cluster{u32, u32}[] [{0, 0}, {6618880, 12369084}]) -> ()  [unwired: 2 in, 2 out]
  n447 = property on="Tab Control" class="TabCtl (strict)"() -> ("Pages"=w1:refnum<vi>[])  [unwired: 2 in, 2 out]
  n448 = property on="Tab Control" class="TabCtl (strict)"() -> ("Pages"=w20:refnum<vi>[])  [unwired: 2 in, 2 out]
  n449 = property on="Tab Control" class="TabCtl (strict)"() -> ("Pages"=w13:refnum<vi>[])  [unwired: 2 in, 2 out]
  n450 = property on="Tab Control" class="TabCtl (strict)"() -> ("Pages"=w5:refnum<vi>[])  [unwired: 2 in, 2 out]
  n451 = property on="Tab Control" class="TabCtl (strict)"() -> ("Pages"=w12:refnum<vi>[])  [unwired: 2 in, 2 out]
  n452 = Index Array(array=w1, index=5) -> (element=w3:refnum<vi>)
  n453 = Index Array "Index Array"(array=w20, index=1) -> (element=w18:refnum<vi>)
  n454 = Index Array(array=w13, index=2) -> (element=w15:refnum<vi>)
  n455 = Index Array(array=w5, index=3) -> (element=w7:refnum<vi>)
  n456 = Index Array(array=w12, index=4) -> (element=w10:refnum<vi>)
  n457 = property class="Page"(reference=w3, "PageEnb"=T2."Page Disabled & Grayed" ("Page Enabled State")) -> ()  [unwired: 1 in, 2 out]
  n458 = property class="Page"(reference=w18, "PageEnb"=T2."Page Disabled & Grayed" ("Page Enabled State")) -> ()  [unwired: 1 in, 2 out]
  n459 = property class="Page"(reference=w15, "PageEnb"=T2."Page Disabled & Grayed" ("Page Enabled State")) -> ()  [unwired: 1 in, 2 out]
  n460 = property class="Page"(reference=w7, "PageEnb"=T2."Page Disabled & Grayed" ("Page Enabled State")) -> ()  [unwired: 1 in, 2 out]
  n461 = property class="Page"(reference=w10, "PageEnb"=T2."Page Disabled & Grayed" ("Page Enabled State")) -> ()  [unwired: 1 in, 2 out]
  n462 = local write "Living Room"(w21) -> ()
  n463 = local write "Laundry 2"(w21) -> ()
  n464 = local write "Bedroom 2"(w21) -> ()
  n465 = local write "Laundry 1"(w21) -> ()
  n466 = local write "Bedroom 1"(w21) -> ()
  n467 = local write "Laundry 3"(w21) -> ()
  n468 = local write "Laundry 4"(w21) -> ()
  n469 = local write "Bathroom 1"(w21) -> ()
  n470 = local write "Bathroom 2"(w21) -> ()
  n471 = local write "Kitchen"(w21) -> ()
  n472 = local write "Dining"(w21) -> ()
  n473 = while {
    stop <- FALSE stop-if-true
    n474 = Get Date/Time In Seconds() -> (seconds since 1Jan1904=→"Time Stamp":timestamp)
    n475 = property on="Time Stamp" class="AbsTime (strict)"("NumText.BGColor"=u32 0 ("Numeric Text.Text Colors:BG Color")) -> ()  [unwired: 2 in, 2 out]
  }
  "Verification" <- FALSE ("Verification")
  "PIN" <- "" ("PIN")
  "Instruction" <- "Enter PIN:" ("Instruction")
  "Login" <- FALSE
